vi "asynchronous process safe state.vi"(9 "Module Info In":T1, 11 "Engine Tags In":T5) -> (1 "Module Info Out":T1, 3 "Engine Tags Out":T5)   [LabVIEW 2013, in "Standard Engine Runtime.lvclass"]
uses:
  Standard Engine Runtime.lvclass
  <vilib>/NI/Tag Bus/table/data table.ctl
  async execution info.ctl
  asynchronous process data.ctl
  async command notification.ctl
  <vilib>/NI/Tag Bus Module Framework/runtime/execution settings.ctl
  async error info.ctl
  <vilib>/NI/Tag Bus Module Framework/runtime/error classification.ctl
  Data Table with Transfer Spec.ctl
  <vilib>/NI/Tag Bus/table/transfer specification.ctl
  <vilib>/NI/Tag Bus/tag/Data Type.ctl
  Configuration/Module Decimation.ctl
  Configuration/Module Error Configuration.ctl
  Configuration/Error Actions By Category.ctl
  Configuration/Error Actions.ctl
  <vilib>/NI/Tag Bus/table/data table.lvlib
  <vilib>/NI/Tag Bus/tag/tag descriptor.lvclass
  Configuration/Standard Engine Configuration.lvclass
  <vilib>/NI/Tag Bus Module Framework/runtime/TBM module execution interface.lvclass
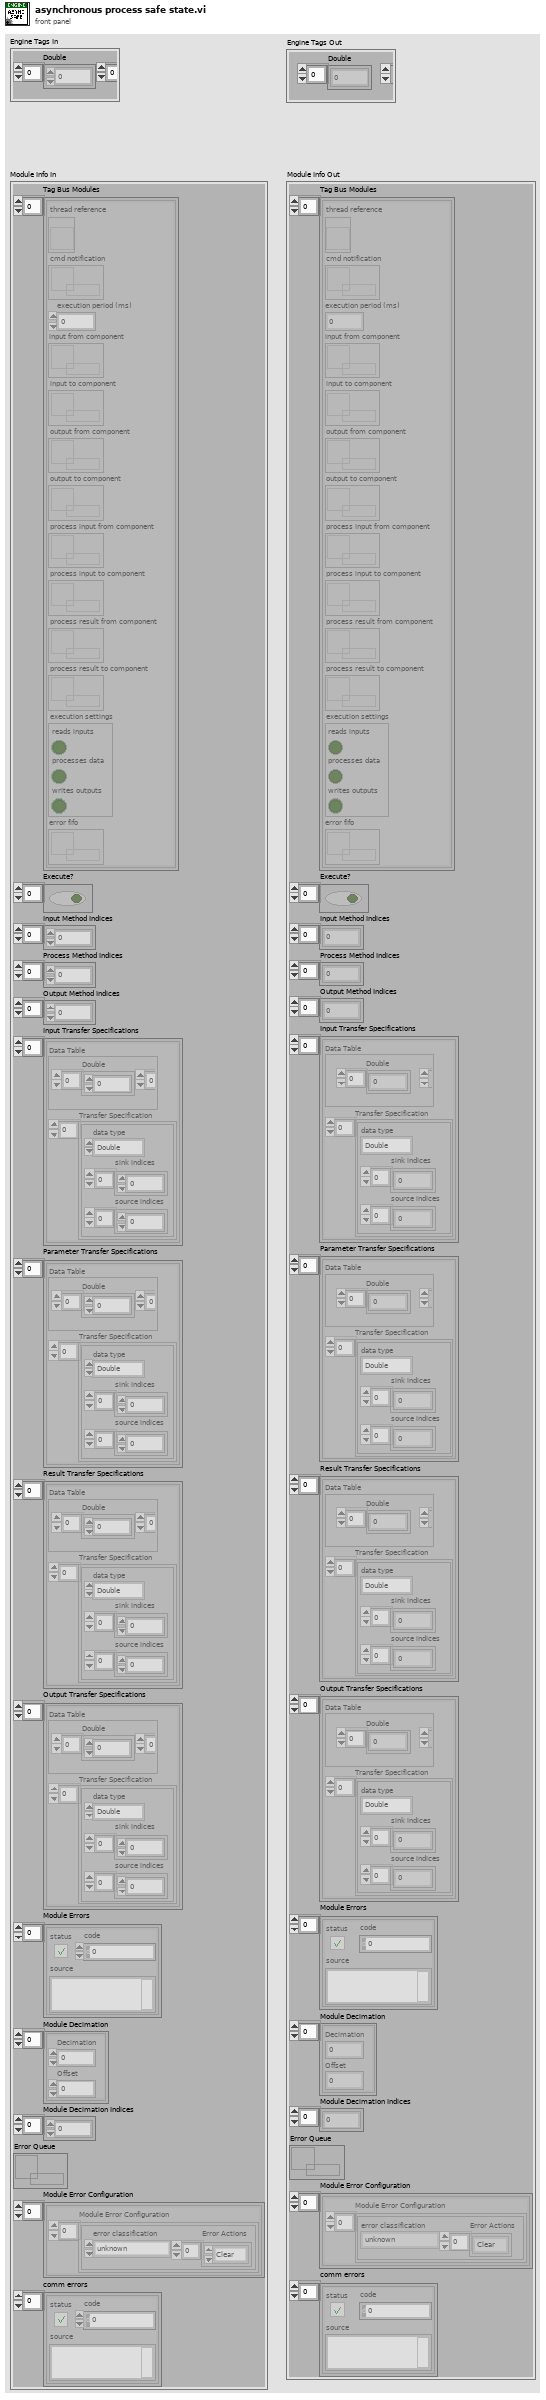
[diagram p1: front panel]
types:
  T1 = typedef "Standard Engine Runtime.lvclass/async execution info.ctl" = cluster{"Tag Bus Modules":T2[], "Execute?":bool[], "Input Method Indices":i32[], "Process Method Indices":i32[], "Output Method Indices":i32[], "Input Transfer Specifications":T4[], "Parameter Transfer Specifications":T4[], "Result Transfer Specifications":T4[], "Output Transfer Specifications":T4[], "Module Errors":errorcluster[], "Module Decimation":T8[], "Module Decimation Indices":i32[], "Error Queue":refnum<queue>, "Module Error Configuration":T9[], "comm errors":errorcluster[]}
  T2 = typedef "Standard Engine Runtime.lvclass/asynchronous process data.ctl" = cluster{"thread reference":refnum<vi>, "cmd notification":refnum<k33>, "execution period (ms)":i32, "input from component":refnum<queue>, "input to component":refnum<queue>, "output from component":refnum<queue>, "output to component":refnum<queue>, "process input from component":refnum<queue>, "process input to component":refnum<queue>, "process result from component":refnum<queue>, "process result to component":refnum<queue>, "execution settings":T3, "error fifo":refnum<k33>}
  T3 = typedef "TBM module execution interface.lvclass/execution settings.ctl" = cluster{"reads inputs":bool, "processes data":bool, "writes outputs":bool}
  T4 = typedef "Standard Engine Runtime.lvclass/Data Table with Transfer Spec.ctl" = cluster{"Data Table":T5, "Transfer Specification":T6[]}
  T5 = typedef "tag bus.lvlib/data table.lvlib/data table.ctl" = cluster{"Double":dbl[], "Single":sgl[], "I64":i64[], "I32":i32[], "I16":i16[], "I8":i8[], "U64":u64[], "U32":u32[], "U16":u16[], "U8":u8[], "Boolean":bool[], "String":string[], "Array of Double":cluster{"DBL Array":dbl[]}[], "Array of Single":cluster{"SGL Array":sgl[]}[], "Array of I64":cluster{"I64 Array":i64[]}[], "Array of I32":cluster{"I32 Array":i32[]}[], "Array of I16":cluster{"I16 Array":i16[]}[], "Array of I8":cluster{"I8 Array":i8[]}[], "Array of U64":cluster{"U64 Array":u64[]}[], "Array of U32":cluster{"U32 Array":u32[]}[], "Array of U16":cluster{"U16 Array":u16[]}[], "Array of U8":cluster{"U8 Array":u8[]}[], "Array of Boolean":cluster{"Boolean Array":bool[]}[], "Array of String":cluster{"String Array":string[]}[]}
  T6 = typedef "tag bus.lvlib/data table.lvlib/transfer specification.ctl" = cluster{"data type":T7, "sink indices":i32[], "source indices":i32[]}
  T7 = typedef "tag bus.lvlib/tag descriptor.lvclass/Data Type.ctl" = enum16{"Double", "Single", "I64", "I32", "I16", "I8", "U64", "U32", "U16", "U8", "Boolean", "String", "Array of Double", "Array of Single", "Array of I64", "Array of I32", "Array of I16", "Array of I8", "Array of U64", "Array of U32", "Array of U16", "Array of U8", "Array of Boolean", "Array of String"}
  T8 = typedef "Standard Engine Configuration.lvclass/Module Decimation.ctl" = cluster{"Decimation":u16, "Offset":u16}
  T9 = typedef "Standard Engine Configuration.lvclass/Module Error Configuration.ctl" = cluster{"Module Error Configuration":T10[]}
  T10 = typedef "Standard Engine Configuration.lvclass/Error Actions By Category.ctl" = cluster{"error classification":T11, "Error Actions":T12[]}
  T11 = typedef "TBM module execution interface.lvclass/error classification.ctl" = enum16{"unknown", "none", "trivial", "recoverable", "critical"}
  T12 = typedef "Standard Engine Configuration.lvclass/Error Actions.ctl" = enum16{"Clear", "Notify", "Stop Component", "Stop Engine", "Safe State", "Attempt Recovery"}
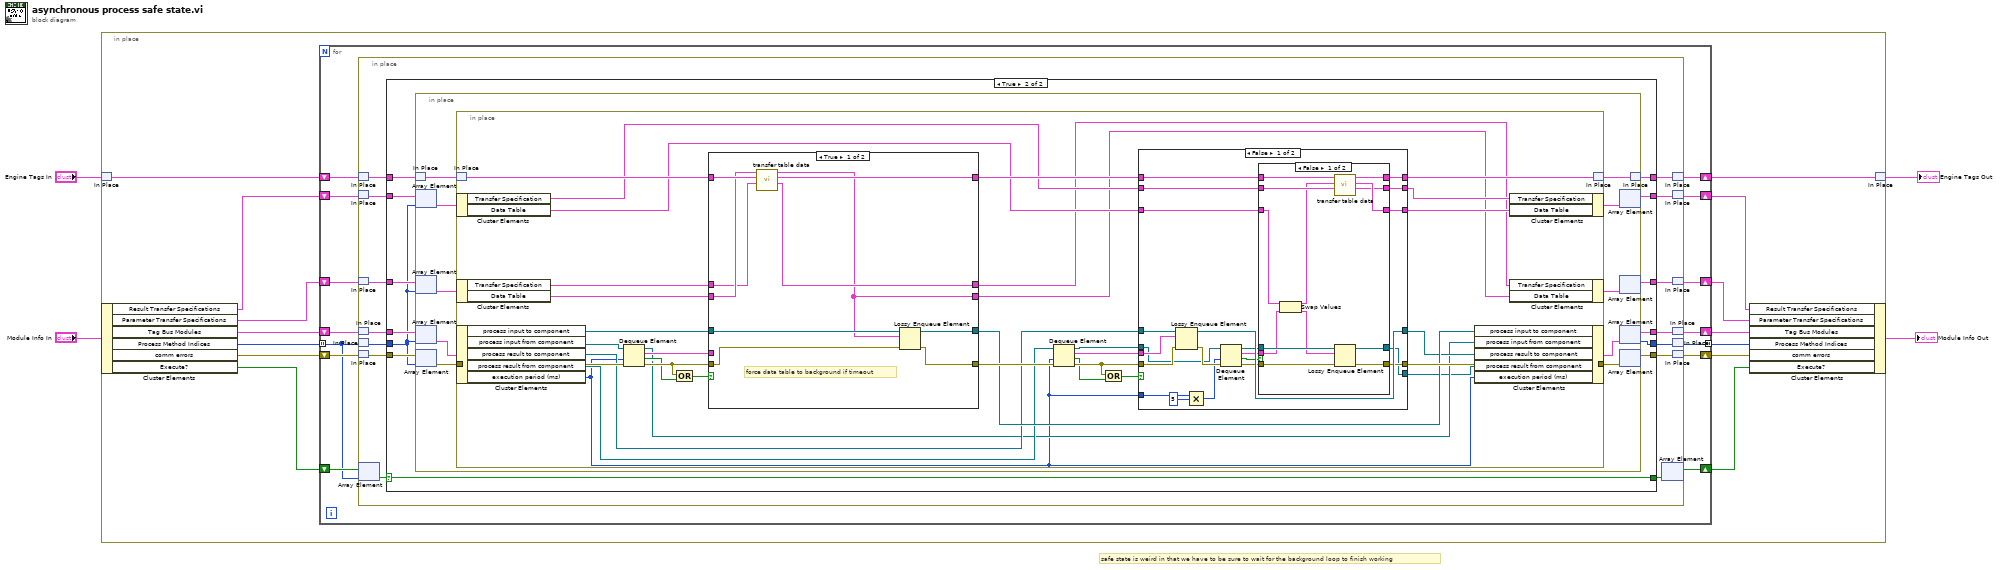
[diagram p0: block diagram]
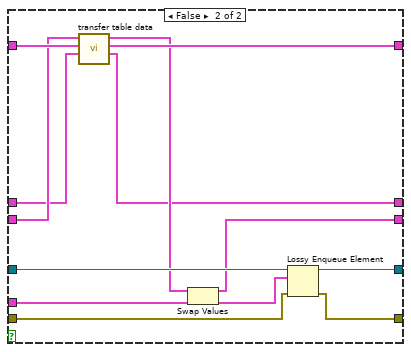
[diagram p5: hidden frame]
diagram:
  # "safe state is weird in that we have to be sure to wait for the background loop to finish working"
  n1 = in-place {
    n2 = in-place-match #1("Engine Tags In") -> (w17:T5)
    n3 = in-place-cluster #2("Module Info In") -> ("Result Transfer Specifications"=w6:T4[], "Parameter Transfer Specifications"=w15:T4[], "Tag Bus Modules"=w12:T2[], "Process Method Indices"=w18:i32[], "comm errors"=w14:errorcluster[], "Execute?"=w8:bool[])
    n4 = for {
      shift-right: [w25] -> w11
      shift-left: w12 -> [w26]
      tunnel: w18 -> [w22] mode=indexing
      shift-right: [w29] -> w16
      shift-left: w17 -> [w30]
      shift-right: [w27] -> w13
      shift-left: w15 -> [w28]
      shift-right: [w23] -> w10
      shift-left: w14 -> [w24]
      tunnel: [w21] -> w9 mode=indexing
      shift-right: [w31] -> w7
      shift-left: w8 -> [w32]
      shift-right: [w19] -> w5
      shift-left: w6 -> [w20]
      n5 = in-place {
        n6 = in-place-match #3(w30) -> (w44:T5)
        n7 = in-place-match #4(w20) -> (w33:T4[])
        n8 = in-place-match #5(w28) -> (w42:T4[])
        n9 = in-place-match #6(w26) -> (w40:T2[])
        n10 = in-place-match #7(w22) -> (w36:i32)
        n11 = in-place-match #8(w24) -> (w38:errorcluster[])
        n12 = in-place-array #9(w32, w22) -> (w46:bool)
        n13 = case shown="True" w46 {
          selector: w46 -> [w48 w57]
          tunnel: w44 -> [w53 w66]
          tunnel: [w53 w65] -> w43
          tunnel: w42 -> [w52 w64]
          tunnel: w40 -> [w51 w63]
          tunnel: w38 -> [w49 w62]
          tunnel: [w52 w61] -> w41
          tunnel: [w49 w60] -> w37
          tunnel: [w51 w59] -> w39
          tunnel: w36 -> [w50 w54]
          tunnel: [w50 w58] -> w35
          tunnel: [w48 w57] -> w45
          tunnel: [w47 w55] -> w34
          tunnel: w33 -> [w47 w56]
          frame False {
          }
          frame True {
            n14 = in-place {
              n15 = in-place-match #10(w66) -> (w76:T5)
              n16 = in-place-array #11(w56, w54) -> (w68:T4)
              n17 = in-place-array #12(w64, w54) -> (w74:T4)
              n18 = in-place-array #13(w63, w54) -> (w72:T2)
              n19 = in-place-array #14(w62, w54) -> (w70:errorcluster)
              n20 = in-place {
                in-place-border: w70 -> [w106]
                in-place-border: [w92] -> w69
                n21 = in-place-match #15(w76) -> (w108:T5)
                n22 = in-place-cluster #16(w68) -> ("Transfer Specification"=w97:T6[], "Data Table"=w94:T5)
                n23 = in-place-cluster #17(w74) -> ("Transfer Specification"=w107:T6[], "Data Table"=w105:T5)
                n24 = in-place-cluster #18(w72) -> ("process input to component"=w104:refnum<queue>, "process input from component"=w103:refnum<queue>, "process result to component"=w87:refnum<queue>, "process result from component"=w88:refnum<queue>, "execution period (ms)"=w77:i32)
                n25 = Dequeue Element(queue=w103, timeout in ms (-1)=w77, error in (no error)=w106) -> (queue out=w84:refnum<queue>, element=w85:T5, timed out?=w86:bool, error out=w101:errorcluster)
                n26 = Compound Arithmetic op=OR(w101, w86) -> (w102:bool)
                n27 = case shown="True" w102 {
                  tunnel: w108 -> [w159 w170]
                  tunnel: [w158 w169] -> w99
                  tunnel: [w154 w172] -> w91
                  tunnel: w107 -> [w156 w166]
                  tunnel: [w155 w165] -> w93
                  tunnel: w105 -> [w157 w168]
                  tunnel: w104 -> [w163 w176]
                  tunnel: [w162 w175] -> w90
                  tunnel: [w161 w174] -> w100
                  tunnel: w101 -> [w160 w173]
                  tunnel: w85 -> [_ w164]
                  frame True {
                    # "force data table to background if timeout"
                    n28 = call <vilib>:"transfer table data.vi"("transfer specification in"=w156, "data table source in"=w159, "data table sink in"=w157) -> ("transfer specification out"=w155:T6[], "data table source out"=w158:T5, "data table sink out"=w154:T5)  [unwired: 6 in]
                    n29 = Lossy Enqueue Element(queue=w163, element=w154, error in (no error)=w160) -> (queue out=w162:refnum<queue>, error out=w161:errorcluster)  [unwired: 2 out]
                  }
                  frame False {
                    n30 = call <vilib>:"transfer table data.vi"("transfer specification in"=w166, "data table source in"=w170, "data table sink in"=w168) -> ("transfer specification out"=w165:T6[], "data table source out"=w169:T5, "data table sink out"=w167:T5)  [unwired: 6 in]
                    n31 = Swap Values(12:w167, 14:w164) -> (1:w172:T5, 3:w171:T5)  [unwired: 1 in]
                    n32 = Lossy Enqueue Element(queue=w176, element=w171, error in (no error)=w173) -> (queue out=w175:refnum<queue>, error out=w174:errorcluster)  [unwired: 2 out]
                  }
                }
                n33 = Dequeue Element(queue=w88, timeout in ms (-1)=w77, error in (no error)=w100) -> (queue out=w79:refnum<queue>, element=w80:T5, timed out?=w81:bool, error out=w82:errorcluster)
                n34 = Compound Arithmetic op=OR(w82, w81) -> (w83:bool)
                n35 = case shown="False" w83 {
                  tunnel: w99 -> [w129 w149]
                  tunnel: [w128 w149] -> w98
                  tunnel: [w127 w151] -> w95
                  tunnel: w97 -> [w126 w150]
                  tunnel: [w125 w150] -> w96
                  tunnel: w94 -> [w124 w151]
                  tunnel: w87 -> [w123 w153]
                  tunnel: [w122 w153] -> w89
                  tunnel: [w112 w152] -> w92
                  tunnel: w82 -> [w120 w152]
                  tunnel: w80 -> [w121 _]
                  tunnel: w79 -> [w118 w148]
                  tunnel: [w111 w148] -> w78
                  tunnel: w77 -> [w117 _]
                  frame False {
                    n36 = Lossy Enqueue Element(queue=w123, element=w121, error in (no error)=w120) -> (queue out=w122:refnum<queue>, error out=w119:errorcluster)  [unwired: 2 out]
                    n37 = Multiply(x=w117, y=5) -> (x*y=w115:i32)
                    n38 = Dequeue Element(queue=w118, timeout in ms (-1)=w115, error in (no error)=w119) -> (queue out=w110:refnum<queue>, element=w109:T5, timed out?=w113:bool, error out=w114:errorcluster)
                    n39 = case shown="False" w113 {
                      tunnel: w129 -> [w142 w145]
                      tunnel: [w141 w145] -> w128
                      tunnel: [w140 w143] -> w127
                      tunnel: w126 -> [w139 w144]
                      tunnel: [w138 w144] -> w125
                      tunnel: w124 -> [w132 w143]
                      tunnel: w114 -> [w137 w147]
                      tunnel: [w136 w147] -> w112
                      tunnel: [w134 w146] -> w111
                      tunnel: w110 -> [w135 w146]
                      tunnel: w109 -> [w133 _]
                      frame False {
                        n40 = Swap Values(12:w132, 14:w133) -> (1:w130:T5, 3:w131:T5)  [unwired: 1 in]
                        n41 = call <vilib>:"transfer table data.vi"("transfer specification in"=w139, "data table source in"=w130, "data table sink in"=w142) -> ("transfer specification out"=w138:T6[], "data table source out"=w140:T5, "data table sink out"=w141:T5)  [unwired: 6 in]
                        n42 = Lossy Enqueue Element(queue=w135, element=w131, error in (no error)=w137) -> (queue out=w134:refnum<queue>, error out=w136:errorcluster)  [unwired: 2 out]
                      }
                      frame True {
                      }
                    }
                  }
                  frame True {
                  }
                }
                n43 = in-place-cluster #18("process input to component"=w90, "process input from component"=w84, "process result to component"=w89, "process result from component"=w78, "execution period (ms)"=w77) -> (w71:T2)
                n44 = in-place-cluster #16("Transfer Specification"=w96, "Data Table"=w95) -> (w67:T4)
                n45 = in-place-cluster #17("Transfer Specification"=w93, "Data Table"=w91) -> (w73:T4)
                n46 = in-place-match #15(w98) -> (w75:T5)
              }
              n47 = in-place-array #11(w67) -> (w55:T4[])  [unwired: 1 out]
              n48 = in-place-array #12(w73) -> (w61:T4[])  [unwired: 1 out]
              n49 = in-place-array #13(w71) -> (w59:T2[], w58:i32)
              n50 = in-place-array #14(w69) -> (w60:errorcluster[])  [unwired: 1 out]
              n51 = in-place-match #10(w75) -> (w65:T5)
            }
          }
        }
        n52 = in-place-array #9(w45) -> (w31:bool[])  [unwired: 1 out]
        n53 = in-place-match #3(w43) -> (w29:T5)
        n54 = in-place-match #4(w34) -> (w19:T4[])
        n55 = in-place-match #5(w41) -> (w27:T4[])
        n56 = in-place-match #6(w39) -> (w25:T2[])
        n57 = in-place-match #7(w35) -> (w21:i32)
        n58 = in-place-match #8(w37) -> (w23:errorcluster[])
      }
    }
    n59 = in-place-cluster #2("Result Transfer Specifications"=w5, "Parameter Transfer Specifications"=w13, "Tag Bus Modules"=w11, "Process Method Indices"=w9, "comm errors"=w10, "Execute?"=w7) -> (→"Module Info Out":T1)
    n60 = in-place-match #1(w16) -> (→"Engine Tags Out":T5)
  }
